vi "ButtonPickupLyingDownBarrel.vi"(11 "POVs":i16[](array[numeric])) -> ()   [LabVIEW 2014]
uses:
  PickupRecycleBinLyingDownEnum.ctl
  Gantry/GantryGlobals.vi
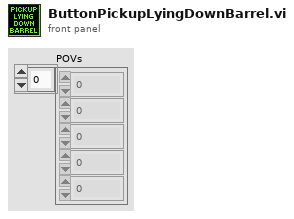
[diagram p1: front panel]
types:
  T1 = typedef "PickupRecycleBinLyingDownEnum.ctl" = enum16{"WaitForInput", "GantryOut", "LiftDown", "Clamp", "LiftUp", "GantryIn"}
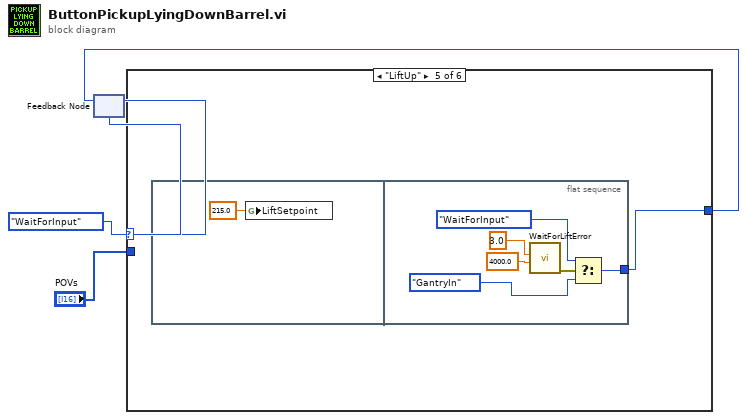
[diagram p0: block diagram]
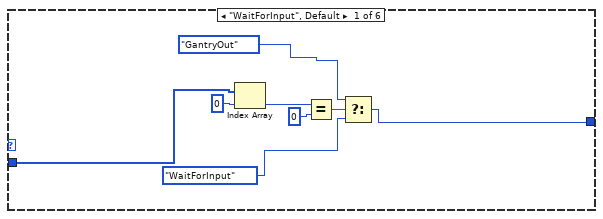
[diagram p2: hidden frame]
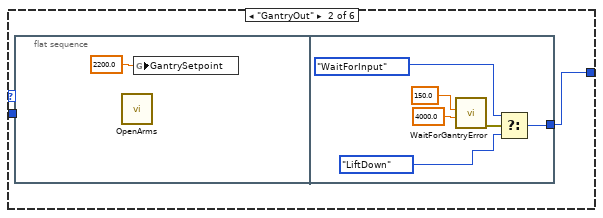
[diagram p3: hidden frame]
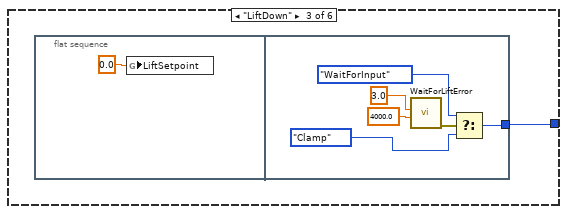
[diagram p4: hidden frame]
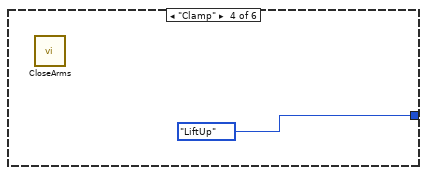
[diagram p5: hidden frame]
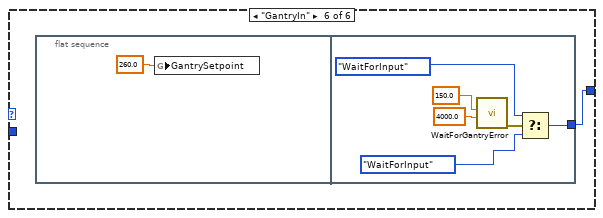
[diagram p6: hidden frame]
diagram:
  n1 = feedback #1(PickupRecycleBinLyingDownEnum."WaitForInput" ("Enum")) -> (w3:T1)
  n2 = case shown="\"LiftUp\"" w3 {
    tunnel: [w8 w13 w21 PickupRecycleBinLyingDownEnum."LiftUp" ("Enum") w30 w38] -> w2
    tunnel: "POVs" -> [w5 _ _ _ _ _]
    frame "WaitForInput", Default {
      n3 = Index Array(array=w5, index=0) -> (element=w11:i16)
      n4 = Equal?(x=w11, y=i16 0) -> (x = y?=w9:bool)
      n5 = Select(t=PickupRecycleBinLyingDownEnum."GantryOut" ("Enum"), s=w9, f=PickupRecycleBinLyingDownEnum."WaitForInput" ("Enum")) -> (s? t:f=w8:T1)
    }
    frame "GantryOut" {
      n6 = flat-sequence {
        tunnel: [w17] -> w13
        frame #0 {
          n7 = call "OpenArms.vi"() -> ()  [unwired: 12 in]
          n8 = global write "GantryGlobals.vi" "GantrySetpoint"(2200.0 ("GantrySetpoint")) -> ()
        }
        frame #1 {
          n9 = call "WaitForGantryError.vi"("Timeout (ms)"=4000.0, "AllowedError"=150.0) -> ("error out"=w18:errorcluster)  [unwired: 9 in]
          n10 = Select(t=PickupRecycleBinLyingDownEnum."WaitForInput" ("Enum"), s=w18, f=PickupRecycleBinLyingDownEnum."LiftDown" ("Enum")) -> (s? t:f=w17:T1)
        }
      }
    }
    frame "LiftDown" {
      n11 = flat-sequence {
        tunnel: [w25] -> w21
        frame #0 {
          n12 = global write "GantryGlobals.vi" "LiftSetpoint"(0.0 ("LiftSetpoint")) -> ()
        }
        frame #1 {
          n13 = call "WaitForLiftError.vi"("Timeout (ms)"=4000.0, "AllowedError"=3.0) -> ("error out"=w28:errorcluster)  [unwired: 9 in]
          n14 = Select(t=PickupRecycleBinLyingDownEnum."WaitForInput" ("Enum"), s=w28, f=PickupRecycleBinLyingDownEnum."Clamp" ("Enum")) -> (s? t:f=w25:T1)
        }
      }
    }
    frame "Clamp" {
      n15 = call "CloseArms.vi"() -> ()  [unwired: 12 in]
    }
    frame "LiftUp" {
      n16 = flat-sequence {
        tunnel: [w34] -> w30
        frame #0 {
          n17 = global write "GantryGlobals.vi" "LiftSetpoint"(215.0 ("LiftSetpoint")) -> ()
        }
        frame #1 {
          n18 = call "WaitForLiftError.vi"("Timeout (ms)"=4000.0, "AllowedError"=3.0) -> ("error out"=w37:errorcluster)  [unwired: 9 in]
          n19 = Select(t=PickupRecycleBinLyingDownEnum."WaitForInput" ("Enum"), s=w37, f=PickupRecycleBinLyingDownEnum."GantryIn" ("Enum")) -> (s? t:f=w34:T1)
        }
      }
    }
    frame "GantryIn" {
      n20 = flat-sequence {
        tunnel: [w42] -> w38
        frame #0 {
          n21 = global write "GantryGlobals.vi" "GantrySetpoint"(260.0 ("GantrySetpoint")) -> ()
        }
        frame #1 {
          n22 = call "WaitForGantryError.vi"("Timeout (ms)"=4000.0, "AllowedError"=150.0) -> ("error out"=w43:errorcluster)  [unwired: 9 in]
          n23 = Select(t=PickupRecycleBinLyingDownEnum."WaitForInput" ("Enum"), s=w43, f=PickupRecycleBinLyingDownEnum."WaitForInput" ("Enum")) -> (s? t:f=w42:T1)
        }
      }
    }
  }
  n24 = feedback-in #1(w2) -> ()
